vi "Get Name.vi"(8 "error in":errorcluster, 11 "Handler in":refnum<class "Handler.lvclass">) -> (0 "error out":errorcluster, 2 "Name":string, 3 "Handler out":refnum<class "Handler.lvclass">)   [LabVIEW 2020, in "hse-logger.lvlib" / "Handler.lvclass"]
doc: "Returns the ``Name`` of the Handler.\n\n____\nHAMPEL SOFTWARE ENGINEERING v2.0.6 (2021-04-15 11:38)"
uses:
  Handler.lvclass
  Handler.lvclass/Handler.ctl
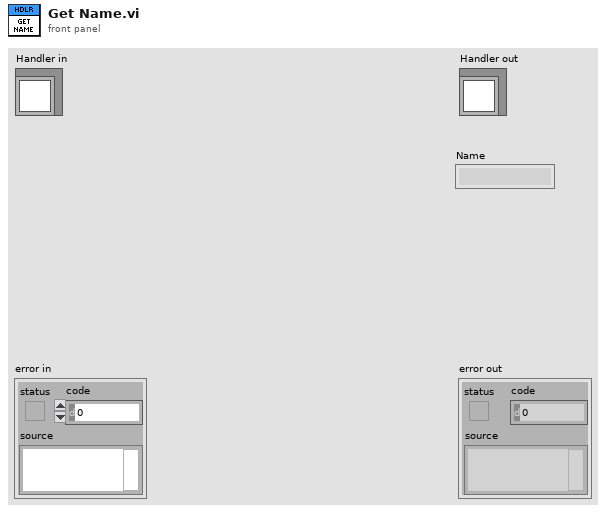
[diagram p1: front panel]
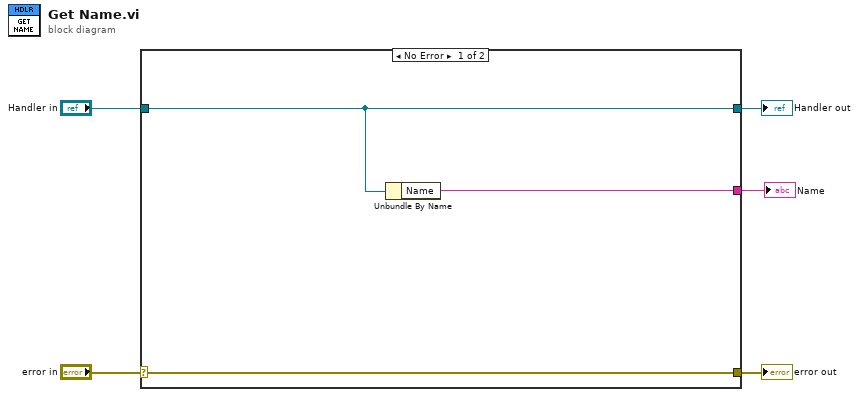
[diagram p0: block diagram]
diagram:
  n1 = case shown="No Error" "error in" {
    selector: "error in" -> [w8 w10]
    tunnel: [w8 w10] -> w4
    tunnel: [w7 w9] -> w2
    tunnel: "Handler in" -> [w7 w9]
    tunnel: [w6 _] -> w1
    frame No Error {
      n2 = Unbundle By Name(w7) -> ("Name"=w6:string)
    }
    frame Error {
    }
  }
  "error out" <- w4
  "Handler out" <- w2
  "Name" <- w1
